vi "Is Closed.vi"(11 "Lossless in":refnum<class "Lossless.lvclass">) -> (2 "Is Closed?":bool)   [LabVIEW 2022 SP3, in "Enclave.lvlib" / "Lossless.lvclass"]
uses:
  Lossless.lvclass
  Lossless.lvclass/Lossless.ctl
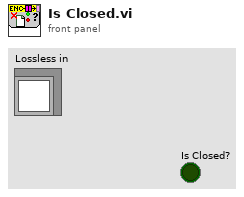
[diagram p1: front panel]
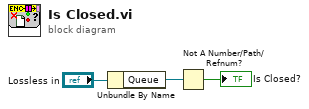
[diagram p0: block diagram]
diagram:
  n1 = Unbundle By Name("Lossless in") -> ("Queue"=w2:refnum<queue>)
  n2 = Not A Number/Path/Refnum?(number/path/refnum=w2) -> (NaN/Path/Refnum?=→"Is Closed?":bool)
